vi "IRead Dew Point DBL.vi"(8 "error in":errorcluster, 10 "Source":string, 11 "IRead Dew Point in":refnum<class "IRead Dew Point.lvclass">) -> (0 "error out":errorcluster, 1 "Time Stamp":timestamp format="%<%x %.3X>T", 2 "Dew Point":dbl, 3 "IRead Dew Point out":refnum<class "IRead Dew Point.lvclass">)   [LabVIEW 2024, in "IRead Dew Point.lvclass"]
uses:
  IRead Dew Point.lvclass
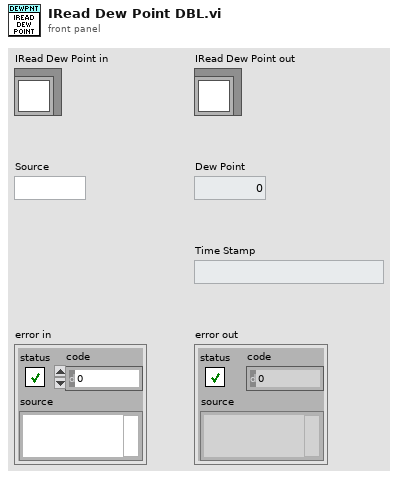
[diagram p1: front panel]
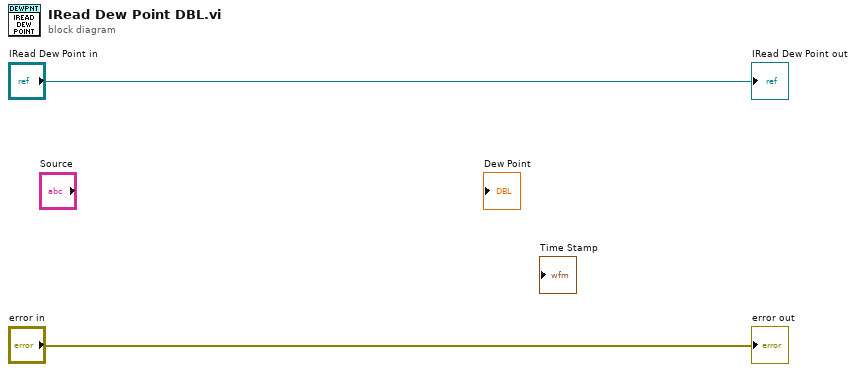
[diagram p0: block diagram]
diagram:
  "error out" <- "error in"
  "IRead Dew Point out" <- "IRead Dew Point in"
